vi "FocusItem.vi"(8 "error in (no error)":errorcluster, 9 "Focus?(False)":bool, 10 "Index":u32, 11 "AdvanceTable in":refnum<class "AdvanceTable.lvclass">) -> (0 "error out":errorcluster, 3 "AdvanceTable out":refnum<class "AdvanceTable.lvclass">)   [LabVIEW 2015, in "ActorManagement.lvlib" / "AdvanceTable.lvclass"]
uses:
  AdvanceTable.lvclass
  AdvanceTable.lvclass/AdvanceTable.ctl
  TableItem/TableItem.lvclass
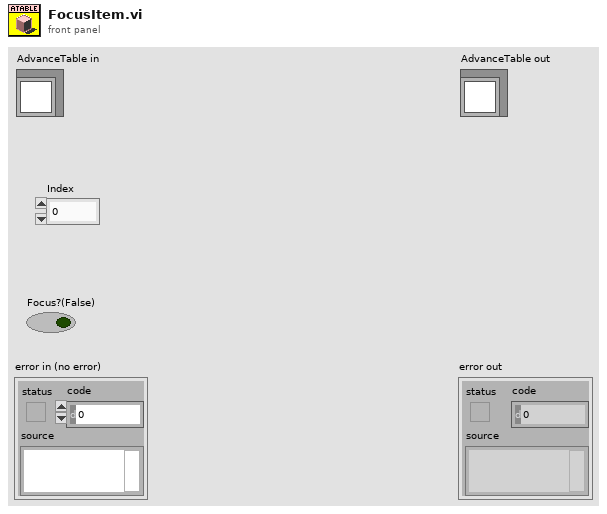
[diagram p1: front panel]
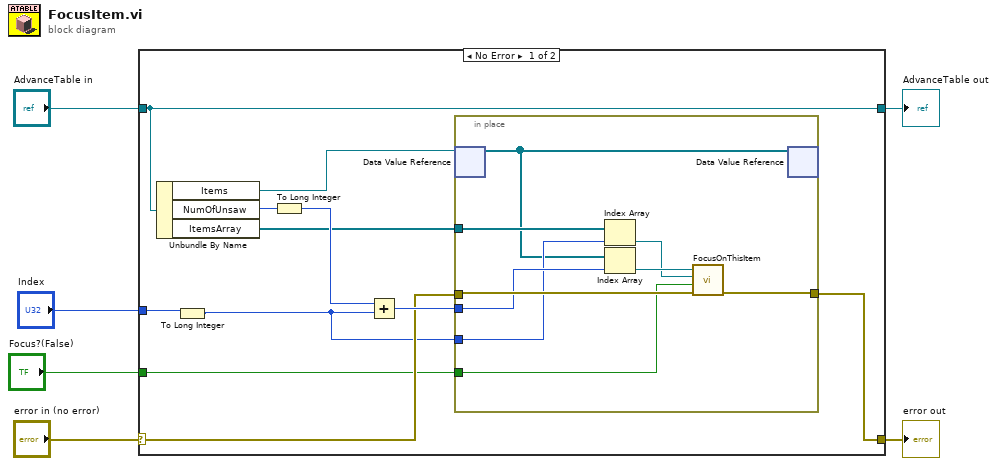
[diagram p0: block diagram]
diagram:
  n1 = case shown="No Error" "error in (no error)" {
    selector: "error in (no error)" -> [w15 w28]
    tunnel: [w14 w28] -> w5
    tunnel: [w17 w27] -> w3
    tunnel: "AdvanceTable in" -> [w17 w27]
    tunnel: "Index" -> [w10 _]
    tunnel: "Focus?(False)" -> [w7 _]
    frame No Error {
      n2 = Unbundle By Name(w17) -> ("Items"=w13:refnum<data-value>, "NumOfUnsaw"=w12:u32, "ItemsArray"=w9:refnum<vi>[])
      n3 = To Long Integer(number=w10) -> (32bit integer=w8:i32)
      n4 = To Long Integer(number=w12) -> (32bit integer=w11:i32)
      n5 = Add(x=w11, y=w8) -> (x+y=w16:i32)
      n6 = in-place {
        in-place-border: w16 -> [w21]
        in-place-border: w15 -> [w26]
        in-place-border: [w25] -> w14
        in-place-border: w9 -> [w24]
        in-place-border: w8 -> [w20]
        in-place-border: w7 -> [w18]
        n7 = in-place-dvr #1(w13) -> (w19:refnum<class "TableItem.lvclass">[])  [unwired: 1 out]
        n8 = Index Array(array=w24, index=w20) -> (element=w22:refnum<vi>)
        n9 = Index Array(array=w19, index=w21) -> (element=w23:refnum<class "TableItem.lvclass">)
        n10 = call-dynamic "FocusOnThisItem.vi"("error in (no error)"=w26, "Focus?(False)"=w18, "ItemCtlRef"=w22, "TableItem in"=w23) -> ("error out"=w25:errorcluster)  [unwired: 6 in, 1 out]
        n11 = in-place-dvr #1(w19) -> ()  [unwired: 2 out]
      }
    }
    frame Error {
    }
  }
  "error out" <- w5
  "AdvanceTable out" <- w3
